vi "空载试验判定.vi"(7 "Result":refnum<vi>, 10 "判定参数":T1, 11 "XY曲线":cluster{"X":dbl[], "Y":dbl[]}[](array[cluster])) -> (2 "判定项长度":i32, 3 "OK？":bool)   [LabVIEW 2019]
uses:
  <userlib>/_MGI/1D Array/MGI Average/MGI Average (DBL[]).vi
panel:
  out "逆向平均值":dbl
  out "正向平均值":dbl
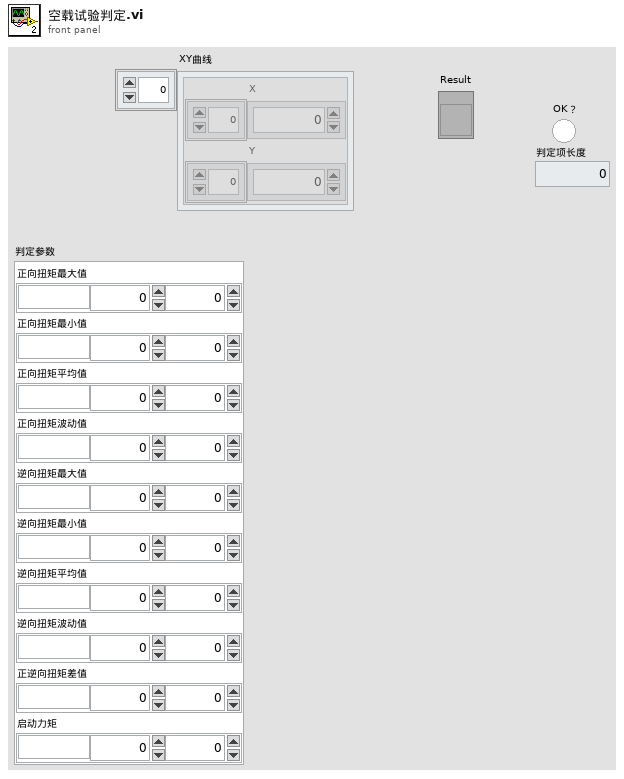
[diagram p1: front panel]
types:
  T1 = cluster{"正向扭矩最大值":cluster{"单位":string, "下限":dbl, "上限":dbl}, "正向扭矩最小值":cluster{"单位":string, "下限":dbl, "上限":dbl}, "正向扭矩平均值":cluster{"单位":string, "下限":dbl, "上限":dbl}, "正向扭矩波动值":cluster{"单位":string, "下限":dbl, "上限":dbl}, "逆向扭矩最大值":cluster{"单位":string, "下限":dbl, "上限":dbl}, "逆向扭矩最小值":cluster{"单位":string, "下限":dbl, "上限":dbl}, "逆向扭矩平均值":cluster{"单位":string, "下限":dbl, "上限":dbl}, "逆向扭矩波动值":cluster{"单位":string, "下限":dbl, "上限":dbl}, "正逆向扭矩差值":cluster{"单位":string, "下限":dbl, "上限":dbl}, "启动力矩":cluster{"单位":string, "下限":dbl, "上限":dbl}}
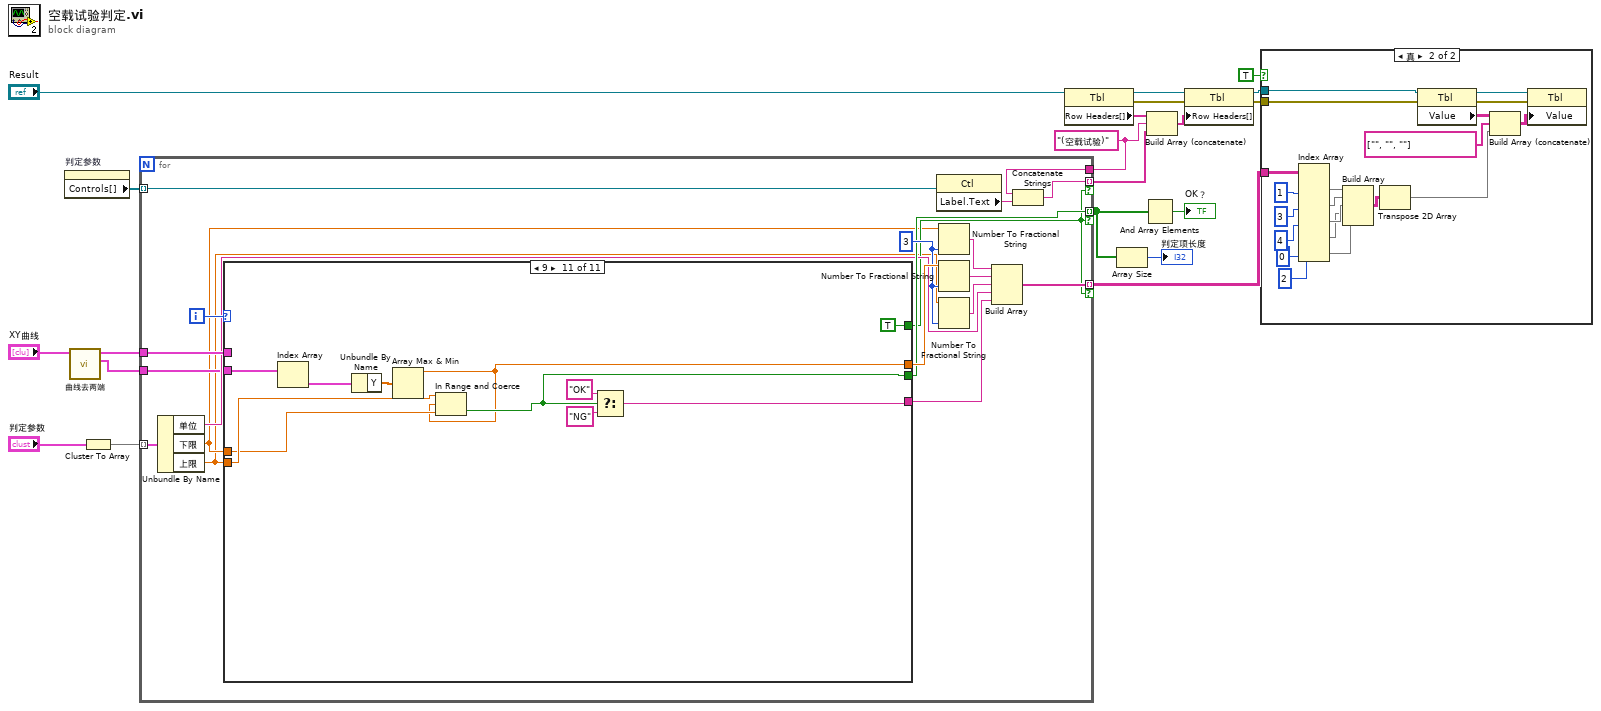
[diagram p0: block diagram]
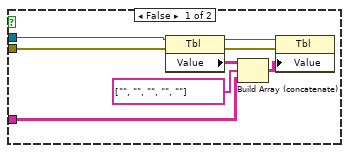
[diagram p2: hidden frame]
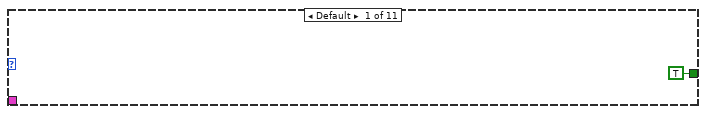
[diagram p3: hidden frame]
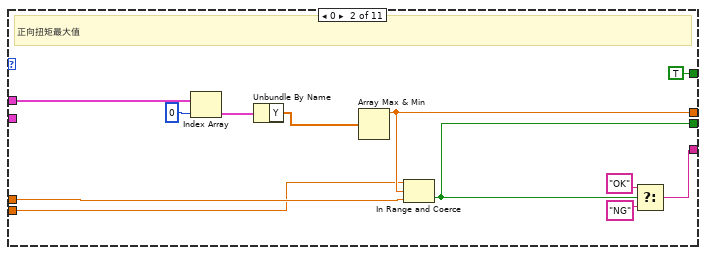
[diagram p4: hidden frame]
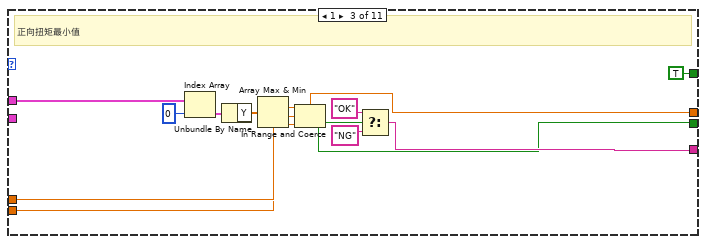
[diagram p5: hidden frame]
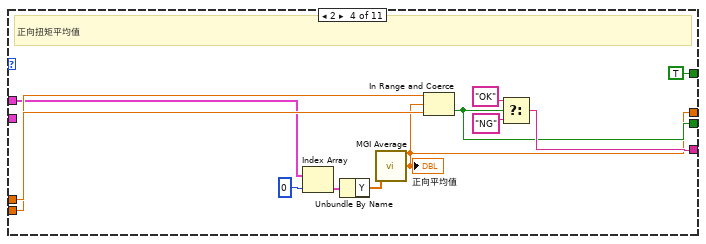
[diagram p6: hidden frame]
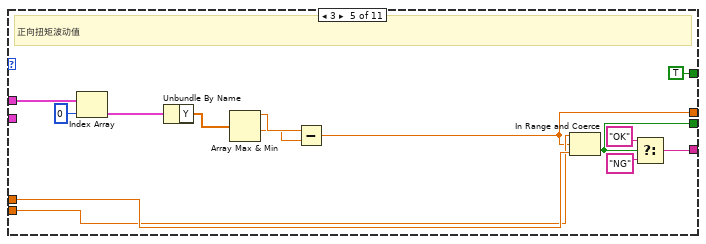
[diagram p7: hidden frame]
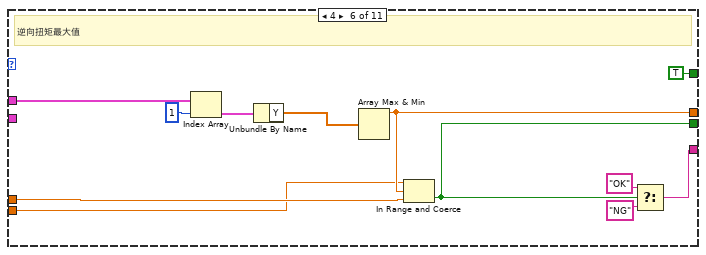
[diagram p8: hidden frame]
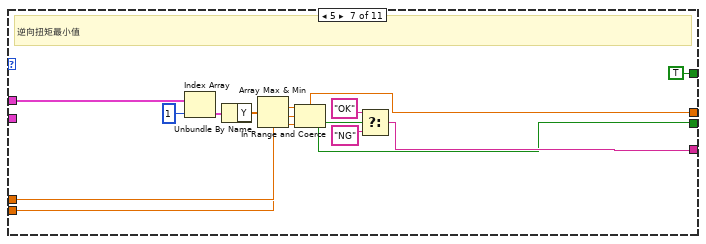
[diagram p9: hidden frame]
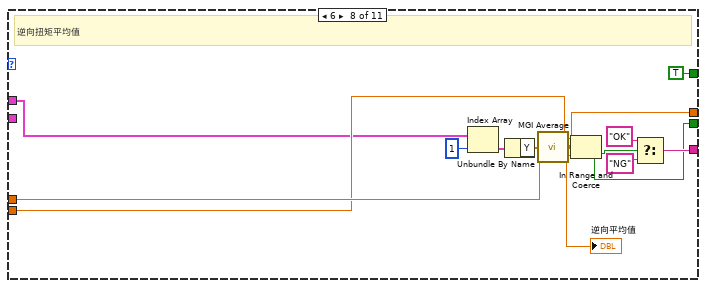
[diagram p10: hidden frame]
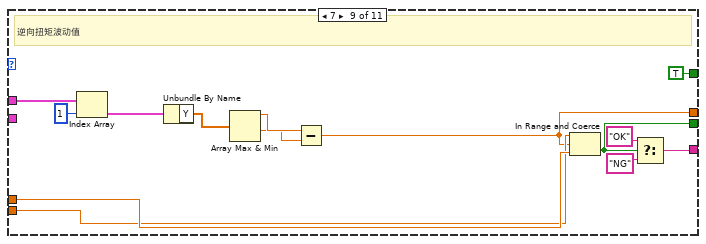
[diagram p11: hidden frame]
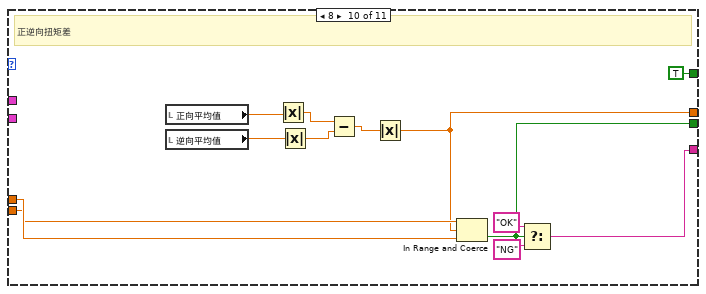
[diagram p12: hidden frame]
diagram:
  w1 = "(空载试验)" ("Label.Text")
  n1 = property on="判定参数" class="Clust (严格)"() -> ("Controls[]"=w9:refnum<vi>[])  [unwired: 2 in, 2 out]
  n2 = call "曲线去两端.vi"("曲线In"="XY曲线") -> ("启动曲线"=w2:cluster{"X":dbl[], "Y":dbl[]}[], "曲线Out"=w5:cluster{"X":dbl[], "Y":dbl[]}[])  [unwired: 9 in]
  n3 = Cluster To Array(cluster="判定参数") -> (array=w20:cluster{"单位":string, "下限":dbl, "上限":dbl}[])
  n4 = for {
    tunnel: w20 -> [w40] mode=indexing
    tunnel: w9 -> [w38] mode=indexing
    tunnel: w5 -> [w36]
    tunnel: [w30] -> w4 mode=indexing if=w26
    tunnel: [w28] -> w10 mode=indexing if=w26
    tunnel: [w22] -> w13 mode=indexing if=w26
    tunnel: w2 -> [w25]
    tunnel: w1 -> [w21]
    i -> [w39]
    w35 = i16 3 ("精度(6)")
    n5 = Unbundle By Name(w40) -> ("单位"=w29:string, "下限"=w24:dbl, "上限"=w23:dbl)
    n6 = case shown="9" w39 {
      tunnel: [_ w50 w56 w67 w78 w100 w106 w116 w128 w142 w156] -> w37
      tunnel: w36 -> [_ w53 w65 w70 w84 w103 w115 w120 w134 _ _]
      tunnel: [_ w47 w61 w75 w89 w97 w111 w125 w139 w144 w155] -> w31
      tunnel: [_ w46 w60 w74 w88 w96 w110 w124 w138 w143 w157] -> w30
      tunnel: w24 -> [_ w45 w59 w73 w87 w95 w109 w123 w137 w151 w161]
      tunnel: w23 -> [_ w44 w58 w72 w86 w94 w108 w122 w136 w150 w162]
      tunnel: [TRUE TRUE TRUE TRUE TRUE TRUE TRUE TRUE TRUE TRUE TRUE] -> w26
      tunnel: w25 -> [_ _ _ _ _ _ _ _ _ _ w165]
      frame Default {
      }
      frame 0 {
        # "正向扭矩最大值"
        n7 = Index Array(array=w53, index=0 ("索引")) -> (element=w51:cluster{"X":dbl[], "Y":dbl[]})
        n8 = Unbundle By Name(w51) -> ("Y"=w42:dbl[])
        n9 = Array Max & Min(array=w42) -> (max value=w50:dbl)  [unwired: 3 out]
        n10 = In Range and Coerce(upper limit=w44, x=w50, lower limit=w45) -> (In Range?=w46:bool)  [unwired: 1 out]
        n11 = Select(t="OK", s=w46, f="NG") -> (s? t:f=w47:string)
      }
      frame 1 {
        # "正向扭矩最小值"
        n12 = Index Array(array=w65, index=0 ("索引")) -> (element=w64:cluster{"X":dbl[], "Y":dbl[]})
        n13 = Unbundle By Name(w64) -> ("Y"=w55:dbl[])
        n14 = Array Max & Min(array=w55) -> (min value=w56:dbl)  [unwired: 3 out]
        n15 = In Range and Coerce(upper limit=w58, x=w56, lower limit=w59) -> (In Range?=w60:bool)  [unwired: 1 out]
        n16 = Select(t="OK", s=w60, f="NG") -> (s? t:f=w61:string)
      }
      frame 2 {
        # "正向扭矩平均值"
        n17 = Index Array(array=w70, index=0 ("索引")) -> (element=w69:cluster{"X":dbl[], "Y":dbl[]})
        n18 = Unbundle By Name(w69) -> ("Y"=w66:dbl[])
        n19 = call-poly <userlib>:"MGI Average.vi"("Double[]"=w66) -> ("Average"=w67:dbl)  [unwired: 1 in]
        "正向平均值" <- w67
        n20 = In Range and Coerce(upper limit=w72, x=w67, lower limit=w73) -> (In Range?=w74:bool)  [unwired: 1 out]
        n21 = Select(t="OK", s=w74, f="NG") -> (s? t:f=w75:string)
      }
      frame 3 {
        # "正向扭矩波动值"
        n22 = Index Array(array=w84, index=0 ("索引")) -> (element=w83:cluster{"X":dbl[], "Y":dbl[]})
        n23 = Unbundle By Name(w83) -> ("Y"=w81:dbl[])
        n24 = Array Max & Min(array=w81) -> (max value=w80:dbl, min value=w79:dbl)  [unwired: 2 out]
        n25 = Subtract(x=w80, y=w79) -> (x-y=w78:dbl)
        n26 = In Range and Coerce(upper limit=w86, x=w78, lower limit=w87) -> (In Range?=w88:bool)  [unwired: 1 out]
        n27 = Select(t="OK", s=w88, f="NG") -> (s? t:f=w89:string)
      }
      frame 4 {
        # "逆向扭矩最大值"
        n28 = Index Array(array=w103, index=1 ("索引")) -> (element=w101:cluster{"X":dbl[], "Y":dbl[]})
        n29 = Unbundle By Name(w101) -> ("Y"=w92:dbl[])
        n30 = Array Max & Min(array=w92) -> (max value=w100:dbl)  [unwired: 3 out]
        n31 = In Range and Coerce(upper limit=w94, x=w100, lower limit=w95) -> (In Range?=w96:bool)  [unwired: 1 out]
        n32 = Select(t="OK", s=w96, f="NG") -> (s? t:f=w97:string)
      }
      frame 5 {
        # "逆向扭矩最小值"
        n33 = Index Array(array=w115, index=1 ("索引")) -> (element=w114:cluster{"X":dbl[], "Y":dbl[]})
        n34 = Unbundle By Name(w114) -> ("Y"=w105:dbl[])
        n35 = Array Max & Min(array=w105) -> (min value=w106:dbl)  [unwired: 3 out]
        n36 = In Range and Coerce(upper limit=w108, x=w106, lower limit=w109) -> (In Range?=w110:bool)  [unwired: 1 out]
        n37 = Select(t="OK", s=w110, f="NG") -> (s? t:f=w111:string)
      }
      frame 6 {
        # "逆向扭矩平均值"
        n38 = Index Array(array=w120, index=1 ("索引")) -> (element=w119:cluster{"X":dbl[], "Y":dbl[]})
        n39 = Unbundle By Name(w119) -> ("Y"=w118:dbl[])
        n40 = call-poly <userlib>:"MGI Average.vi"("Double[]"=w118) -> ("Average"=w116:dbl)  [unwired: 1 in]
        "逆向平均值" <- w116
        n41 = In Range and Coerce(upper limit=w122, x=w116, lower limit=w123) -> (In Range?=w124:bool)  [unwired: 1 out]
        n42 = Select(t="OK", s=w124, f="NG") -> (s? t:f=w125:string)
      }
      frame 7 {
        # "逆向扭矩波动值"
        n43 = Index Array(array=w134, index=1 ("索引")) -> (element=w133:cluster{"X":dbl[], "Y":dbl[]})
        n44 = Unbundle By Name(w133) -> ("Y"=w131:dbl[])
        n45 = Array Max & Min(array=w131) -> (max value=w130:dbl, min value=w129:dbl)  [unwired: 2 out]
        n46 = Subtract(x=w130, y=w129) -> (x-y=w128:dbl)
        n47 = In Range and Coerce(upper limit=w136, x=w128, lower limit=w137) -> (In Range?=w138:bool)  [unwired: 1 out]
        n48 = Select(t="OK", s=w138, f="NG") -> (s? t:f=w139:string)
      }
      frame 8 {
        # "正逆向扭矩差"
        n49 = local read "正向平均值"() -> (w149:dbl)
        n50 = local read "逆向平均值"() -> (w148:dbl)
        n51 = Absolute Value(x=w149) -> (abs(x)=w147:dbl)
        n52 = Absolute Value(x=w148) -> (abs(x)=w146:dbl)
        n53 = Subtract(x=w147, y=w146) -> (x-y=w145:dbl)
        n54 = Absolute Value(x=w145) -> (abs(x)=w142:dbl)
        n55 = In Range and Coerce(upper limit=w150, x=w142, lower limit=w151) -> (In Range?=w143:bool)  [unwired: 1 out]
        n56 = Select(t="OK", s=w143, f="NG") -> (s? t:f=w144:string)
      }
      frame 9 {
        n57 = Index Array(array=w165) -> (element=w164:cluster{"X":dbl[], "Y":dbl[]})  [unwired: 1 in]
        n58 = Unbundle By Name(w164) -> ("Y"=w163:dbl[])
        n59 = Array Max & Min(array=w163) -> (max value=w156:dbl)  [unwired: 3 out]
        n60 = In Range and Coerce(upper limit=w162, x=w156, lower limit=w161) -> (In Range?=w157:bool)  [unwired: 1 out]
        n61 = Select(t="OK", s=w157, f="NG") -> (s? t:f=w155:string)
      }
    }
    n62 = property class="Ctl"(reference=w38) -> ("Label.Text"=w27:string)  [unwired: 1 in, 2 out]
    n63 = Number To Fractional String(number=w24, precision (6)=w35) -> (F-format string=w34:string)  [unwired: 2 in]
    n64 = Number To Fractional String(number=w37, precision (6)=w35) -> (F-format string=w33:string)  [unwired: 2 in]
    n65 = Number To Fractional String(number=w23, precision (6)=w35) -> (F-format string=w32:string)  [unwired: 2 in]
    n66 = Build Array(w34, w33, w32, w29, w31) -> (w28:string[])
    n67 = Concatenate Strings(w21, w27) -> (w22:string)
  }
  n68 = property class="Tbl"(reference="Result") -> (reference out=w15:refnum<vi>, error out=w18:errorcluster, "Row Headers[]"=w11:string[])  [unwired: 1 in]
  n69 = Array Size(array=w4) -> (size(s)=→"判定项长度":i32)
  n70 = And Array Elements(Boolean array=w4) -> (logical AND=→"OK？":bool)
  n71 = Build Array (concatenate)(w11, w1, w13) -> (w14:string[])
  n72 = property class="Tbl"(reference=w15, error in=w18, "Row Headers[]"=w14) -> (reference out=w16:refnum<vi>, error out=w17:errorcluster)
  n73 = case shown="真" TRUE {
    tunnel: w17 -> [w171 w191]
    tunnel: w16 -> [w168 w188]
    tunnel: w10 -> [w167 w186]
    frame False {
      n74 = property class="Tbl"(reference=w168, error in=w171) -> (reference out=w169:refnum<vi>, error out=w170:errorcluster, "Value"=w172:string[][])
      n75 = Build Array (concatenate)(w172, string[] ["", "", "", "", ""], w167) -> (w173:string[][])
      n76 = property class="Tbl"(reference=w169, error in=w170, "Value"=w173) -> ()  [unwired: 2 out]
    }
    frame True {
      n77 = Index Array(array=w186, index (col) #1=1 ("禁用的索引 (列)"), index (col) #2=3 ("索引 (列)"), index (col) #3=4 ("索引 (列)"), index (col) #4=0 ("索引 (列)"), index (col) #5=2 ("索引 (列)")) -> (element #1=w182:string[], element #2=w181:string[], element #3=w180:string[], element #4=w175:string[], element #5=w174:string[])  [unwired: 5 in]
      n78 = Build Array(w182, w181, w180, w175, w174) -> (w179:string[][])
      n79 = Transpose 2D Array(2D array=w179) -> (transposed array=w178:string[][])
      n80 = property class="Tbl"(reference=w188, error in=w191) -> (reference out=w189:refnum<vi>, error out=w190:errorcluster, "Value"=w192:string[][])
      n81 = Build Array (concatenate)(w192, string[] ["", "", ""], w178) -> (w193:string[][])
      n82 = property class="Tbl"(reference=w189, error in=w190, "Value"=w193) -> ()  [unwired: 2 out]
    }
  }
